vi "Configure Session.vi"(8 "error in":errorcluster, 11 "Plugin in":refnum<class "Sift TDMS Uploader.lvclass">) -> (0 "error out":errorcluster, 3 "Plugin out":refnum<class "Sift TDMS Uploader.lvclass">)   [LabVIEW 2024, in "Sift TDMS Uploader.lvlib" / "Sift TDMS Uploader.lvclass"]
uses:
  Sift TDMS Uploader.lvclass
  C:/Program Files/National Instruments/LabVIEW 2024/vi.lib/FlexLogger/SDK/PluginSDK.lvlibp/PEFClasses/SDK/Plugin/Plugin.lvclass
  Sift TDMS Uploader.lvclass/Sift TDMS Uploader.ctl
  <vilib>/FlexLogger/SDK/PluginSDK.lvlibp/PEFClasses/SDK/Plugin/ParameterAccess/Read String.vi
  <vilib>/FlexLogger/SDK/PluginSDK.lvlibp/PEFClasses/SDK/Plugin/Plugin.lvclass
  C:/Program Files/National Instruments/LabVIEW 2024/vi.lib/FlexLogger/SDK/PluginSDK.lvlibp/PEFClasses/SDK/Processing Element/Processing Element.lvclass
  C:/Users/Alex luCK/Documents/Projects/sift-labview/plugins/flexlogger/Sift TDMS Uploader/source/Sift TDMS Uploader.lvclass
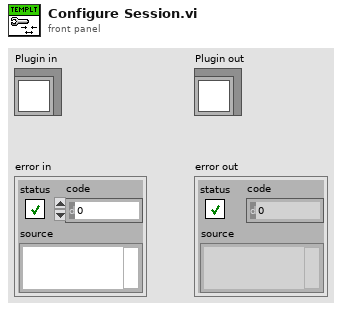
[diagram p1: front panel]
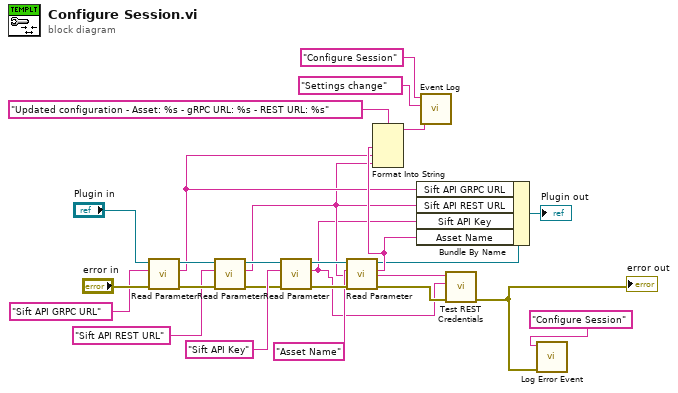
[diagram p0: block diagram]
diagram:
  n1 = call-poly <vilib>:"Read Parameter.vi"("error in (no error)"="error in", "Name"="Sift API GRPC URL", "Plugin in"="Plugin in") -> ("error out"=w14:errorcluster, "Value"=w9:string, "Plugin out"=w15:refnum<class "Sift TDMS Uploader.lvclass">)  [unwired: 5 in, 1 out]
  n2 = call-poly <vilib>:"Read Parameter.vi"("error in (no error)"=w14, "Name"="Sift API REST URL", "Plugin in"=w15) -> ("error out"=w16:errorcluster, "Value"=w2:string, "Plugin out"=w17:refnum<class "Sift TDMS Uploader.lvclass">)  [unwired: 5 in, 1 out]
  n3 = call-poly <vilib>:"Read Parameter.vi"("error in (no error)"=w16, "Name"="Sift API Key", "Plugin in"=w17) -> ("error out"=w25:errorcluster, "Value"=w1:string, "Plugin out"=w24:refnum<class "Sift TDMS Uploader.lvclass">)  [unwired: 5 in, 1 out]
  n4 = call-poly <vilib>:"Read Parameter.vi"("error in (no error)"=w25, "Name"="Asset Name", "Plugin in"=w24) -> ("error out"=w4:errorcluster, "Value"=w10:string, "Plugin out"=w5:refnum<class "Sift TDMS Uploader.lvclass">)  [unwired: 5 in, 1 out]
  n5 = Format Into String(format string="Updated configuration - Asset: %s - gRPC URL: %s - REST URL: %s", w10, w9, w2) -> (resulting string=w8:string)  [unwired: 2 in, 1 out]
  n6 = Bundle By Name(cluster=w5, "Sift API GRPC URL"=w9, "Sift API REST URL"=w2, "Sift API Key"=w1, "Asset Name"=w10) -> (→"Plugin out":refnum<class "Sift TDMS Uploader.lvclass">)
  n7 = call "Event Log.vi"("Message"=w8, "Event Type"="Settings change", "Location"="Configure Session") -> ()  [unwired: 9 in]
  n8 = call "Test REST Credentials.vi"("error in (no error)"=w4, "API Key"=w1, "REST URL"=w2) -> ("error out"=w3:errorcluster)  [unwired: 8 in]
  "error out" <- w3
  n9 = call "Log Error Event.vi"("error in (no error)"=w3, "Location"="Configure Session") -> ()  [unwired: 10 in]
